vi "TOGGLE BOOL.vi"(7 "force":bool, 8 "error in (no error)":errorcluster, 10 "stack ref name":string, 11 "Button Pressed?":bool) -> (0 "error out":errorcluster)   [LabVIEW 2023]
uses:
  <vilib>/Rock Robotics/Network Tables/NT Read Boolean.vi
  <vilib>/Rock Robotics/Network Tables/NT Write Boolean.vi
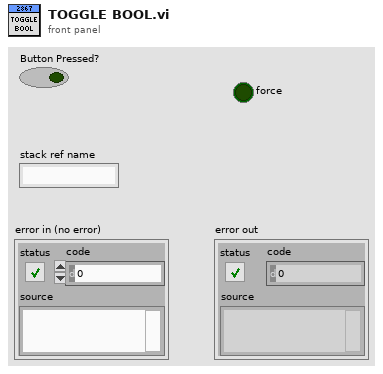
[diagram p1: front panel]
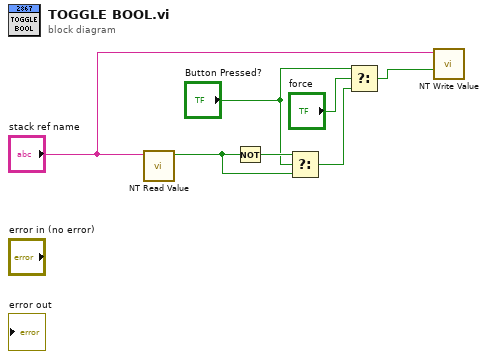
[diagram p0: block diagram]
diagram:
  n1 = call-poly <vilib>:"NT Read Value.vi"("name"="stack ref name") -> ("value"=w6:bool)  [unwired: 8 in, 2 out]
  n2 = Not(x=w6) -> (.not. x?=w7:bool)
  n3 = Select(t=w7, s="Button Pressed?", f=w6) -> (s? t:f=w1:bool)
  n4 = Select(t="Button Pressed?", s="force", f=w1) -> (s? t:f=w4:bool)
  n5 = call-poly <vilib>:"NT Write Value.vi"("value"=w4, "name"="stack ref name") -> ()  [unwired: 9 in, 1 out]
